vi "TestAPI.vi"() -> ()   [LabVIEW 2019, in "Inst.RP100.lvlib" / "Inst.RP100.lvclass"]
uses:
  Inst.RP100.lvclass
  C:/Program Files (x86)/National Instruments/LabVIEW 2019/user.lib/LevyLab/Instrument Framework/Instrument/Instrument.lvclass
  <userlib>/LevyLab/Instrument Framework/Instrument/Instrument.lvclass
panel:
  out "processed data":variant
  in  "index":i32
  out "commands":string[](array[string])
  in  "Instrument?":bool
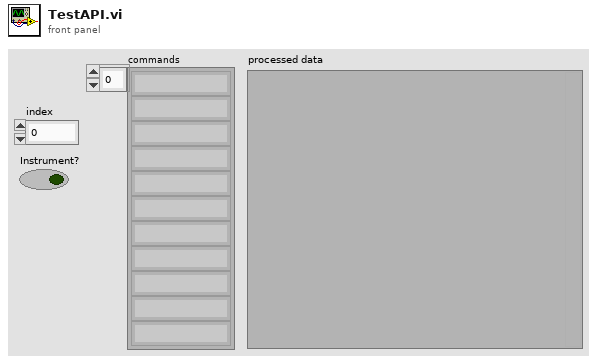
[diagram p1: front panel]
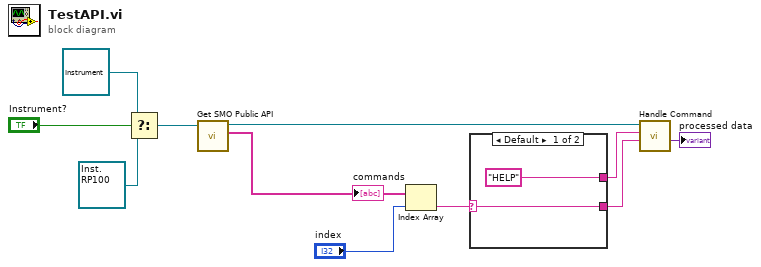
[diagram p0: block diagram]
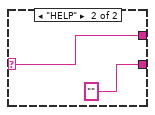
[diagram p2: hidden frame]
diagram:
  n1 = Select(t=refnum<class "Instrument.lvclass"> refnum ("Instrument.lvlib:Instrument.lvclass"), s="Instrument?", f=refnum<class "Inst.RP100.lvclass"> refnum ("Inst.RP100.lvclass")) -> (s? t:f=w2:refnum<class "Instrument.lvclass">)
  n2 = call-dynamic "Get SMO Public API.vi"("Instrument in"=w2) -> ("commands"=w10:string[], "Instrument out"=w4:refnum<class "Instrument.lvclass">)  [unwired: 8 in, 1 out]
  "commands" <- w10
  n3 = Index Array(array=w10, index="index") -> (element=w8:string)
  n4 = case shown="Default" w8 {
    selector: w8 -> [w12 w15]
    tunnel: [w12 ""] -> w5
    tunnel: ["HELP" ("string") w15] -> w6
    frame Default {
    }
    frame "HELP" {
    }
  }
  n5 = call-dynamic "Handle Command.vi"("params in"=w5, "command"=w6, "Instrument in"=w4) -> ("processed data"=→"processed data":variant)  [unwired: 5 in, 3 out]
